vi "ProdaNG.Example.GetLanguages.vi"() -> ()   [LabVIEW 2016]
panel:
  out "Languages":string[](array[string])
  in  "Connection string":string="lcptb/lcptb@PRODA_WPK"
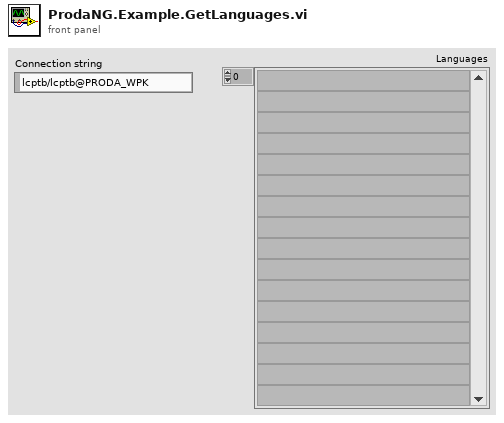
[diagram p1: front panel]
types:
  T1 = typedef "ProdaNG.Language.ctl" = cluster{"i_id":i32, "isoCode":string, "name":string}
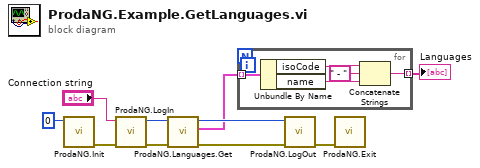
[diagram p0: block diagram]
diagram:
  n1 = call "ProdaNG.Init.vi"("numContexts (0: unlimited)"=0 ("numContexts")) -> ("error out"=w10:errorcluster)  [unwired: 10 in]
  n2 = call "ProdaNG.LogIn.vi"("error in"=w10, "ConnectionString"="Connection string") -> ("error out"=w6:errorcluster, "dbHandle"=w5:i32)  [unwired: 7 in, 1 out]
  n3 = call "ProdaNG.Languages.Get.vi"("error in (no error)"=w6, "dbHandleIn"=w5) -> ("error out"=w4:errorcluster, "Languages"=w2:T1[], "dbHandle"=w3:i32)  [unwired: 7 in]
  n4 = for {
    tunnel: w2 -> [w15] mode=indexing
    tunnel: [w13] -> w1 mode=indexing
    n5 = Unbundle By Name(w15) -> ("isoCode"=w12:string, "name"=w14:string)
    n6 = Concatenate Strings(w12, " - " ("string"), w14) -> (w13:string)
  }
  "Languages" <- w1
  n7 = call "ProdaNG.LogOut.vi"("error in"=w4, "dbHandleIn"=w3) -> ("error out"=w8:errorcluster)  [unwired: 9 in]
  n8 = call "ProdaNG.Exit.vi"("error in (no error)"=w8) -> ()  [unwired: 10 in, 1 out]
